vi "Pre Processing.vi"(0 "pin_map_context":T1, 5 "pin_or_relay_names":string[](array[string]), 11 "error in (no error)":errorcluster) -> (8 "sessions":T2[](array[typedef]), 15 "error out":errorcluster)   [LabVIEW 2024, in "devicePowerSequencerCoreLogic.lvlib"]
uses:
  devicePowerSequencerCoreLogic.lvlib
  <vilib>/Plug-In SDKs/Measurements/Measure Call Context/Measure Call Context.lvclass
  <vilib>/Plug-In SDKs/Measurements/Measure Call Context/Reserve Sessions - NPin.vi
  <vilib>/gRPC/Generated APIs/ni/measurementlink/measurement/v1/RPC Messages/ni_measurementlink_PinMapContext.ctl
  <vilib>/gRPC/Generated APIs/ni/measurementlink/measurement/v1/ni.measurementlink.measurement.v1.api.lvlib
  <vilib>/gRPC/Generated APIs/ni/measurementlink/sessionmanagement/v1/RPC Messages/ni_measurementlink_sessionmanagement_v1_ChannelMapping.ctl
  <vilib>/gRPC/Generated APIs/ni/measurementlink/sessionmanagement/v1/ni.measurementlink.sessionmanagement.v1.api.lvlib
  <vilib>/gRPC/Generated APIs/ni/measurementlink/sessionmanagement/v1/RPC Messages/nidevice_grpc_Session.ctl
  <vilib>/gRPC/Generated APIs/ni/measurementlink/sessionmanagement/v1/RPC Messages/ni_measurementlink_sessionmanagement_v1_SessionInformation.ctl
panel:
  out "measurement context out":refnum<class "Measure Call Context.lvclass">
  in  "measurement context in":refnum<class "Measure Call Context.lvclass">
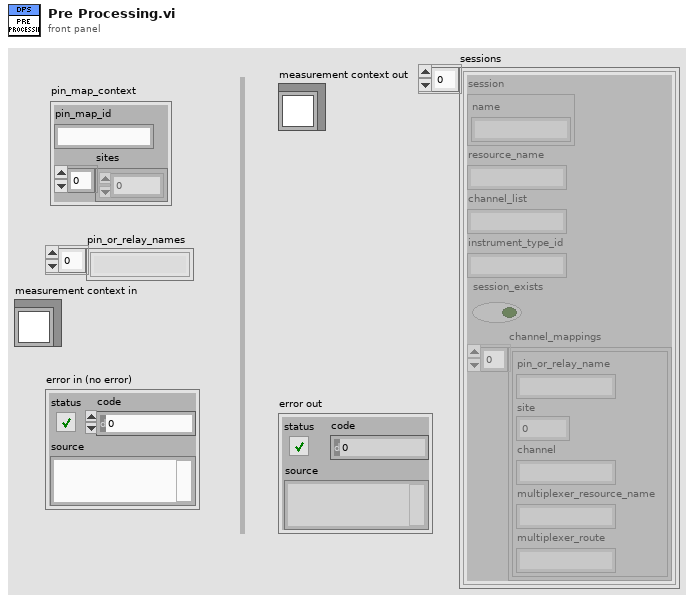
[diagram p1: front panel]
types:
  T1 = typedef "ni.measurementlink.measurement.v1.api.lvlib/ni_measurementlink_PinMapContext.ctl" = cluster{"pin_map_id":string, "sites":i32[]}
  T2 = typedef "ni.measurementlink.sessionmanagement.v1.api.lvlib/ni_measurementlink_sessionmanagement_v1_SessionInformation.ctl" = cluster{"session":T3, "resource_name":string, "channel_list":string, "instrument_type_id":string, "session_exists":bool, "channel_mappings":T4[]}
  T3 = typedef "ni.measurementlink.sessionmanagement.v1.api.lvlib/nidevice_grpc_Session.ctl" = cluster{"name":string}
  T4 = typedef "ni.measurementlink.sessionmanagement.v1.api.lvlib/ni_measurementlink_sessionmanagement_v1_ChannelMapping.ctl" = cluster{"pin_or_relay_name":string, "site":i32, "channel":string, "multiplexer_resource_name":string, "multiplexer_route":string}
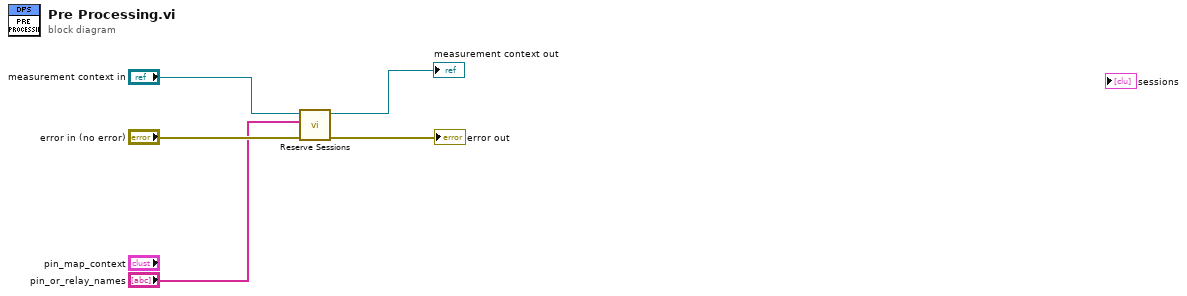
[diagram p0: block diagram]
diagram:
  n1 = call-poly <vilib>:"Reserve Sessions.vi"("error in"="error in (no error)", "pin or relay names"="pin_or_relay_names", "measurement context in"="measurement context in") -> ("error out"=→"error out":errorcluster, "measurement context out"=→"measurement context out":refnum<class "Measure Call Context.lvclass">)  [unwired: 6 in, 1 out]
